vi "Decompose.vi"(0 "object in":refnum<class "Navigation.lvclass">, 2 "value":dbl, 4 "vector":dbl[](array[numeric]), 5 "error in (no error)":errorcluster) -> (14 "object out":refnum<class "Navigation.lvclass">, 16 "xValue":dbl, 18 "yValue":dbl, 19 "error out":errorcluster)   [LabVIEW 2023, in "Navigation.lvclass"]
uses:
  Navigation.lvclass
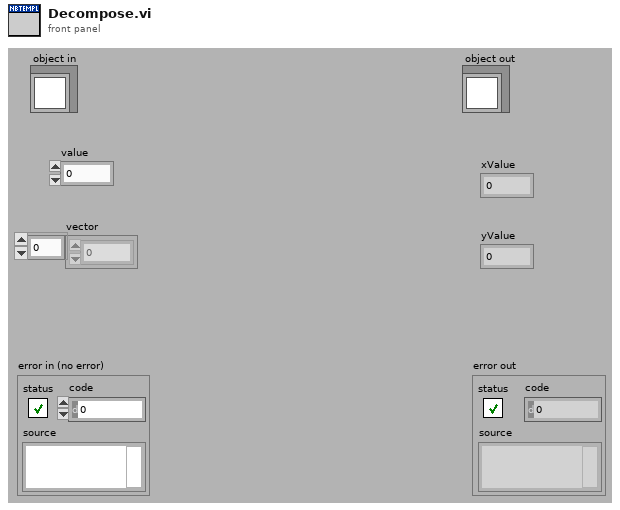
[diagram p1: front panel]
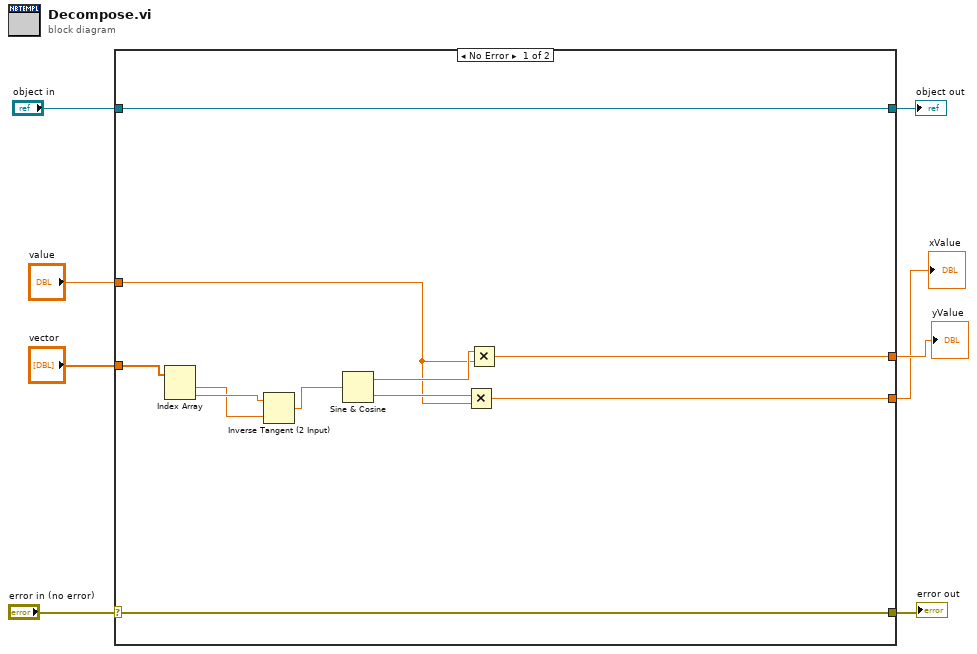
[diagram p0: block diagram]
diagram:
  n1 = case shown="No Error" "error in (no error)" {
    selector: "error in (no error)" -> [w18 w21]
    tunnel: [w18 w21] -> w7
    tunnel: [w19 w20] -> w5
    tunnel: "object in" -> [w19 w20]
    tunnel: "vector" -> [w17 _]
    tunnel: "value" -> [w10 _]
    tunnel: [w12 _] -> w2
    tunnel: [w9 _] -> w1
    frame No Error {
      n2 = Index Array(array=w17) -> (element #1=w15:dbl, element #2=w16:dbl)  [unwired: 2 in]
      n3 = Inverse Tangent (2 Input)(1:w15, 2:w16) -> (0:w14:dbl)
      n4 = Sine & Cosine(0:w14) -> (1:w13:dbl, 2:w11:dbl)
      n5 = Multiply(x=w11, y=w10) -> (x*y=w9:dbl)
      n6 = Multiply(x=w13, y=w10) -> (x*y=w12:dbl)
    }
    frame Error {
    }
  }
  "error out" <- w7
  "object out" <- w5
  "xValue" <- w1
  "yValue" <- w2
